vi "Close Hardware.vi"(8 "error in (no error)":errorcluster, 11 "Instrument.Template in":refnum<class "Instrument.Framework-Template.lvclass">) -> (0 "error out":errorcluster, 3 "Instrument.Template out":refnum<class "Instrument.Framework-Template.lvclass">)   [LabVIEW 2019, in "Instrument.Framework-Template.lvclass"]
uses:
  Instrument.Framework-Template.lvclass
  Instrument.Framework-Template.lvclass/Instrument.Framework-Template.ctl
  Framework/Instrument Types/SCPI/Instrument.SCPI.lvclass
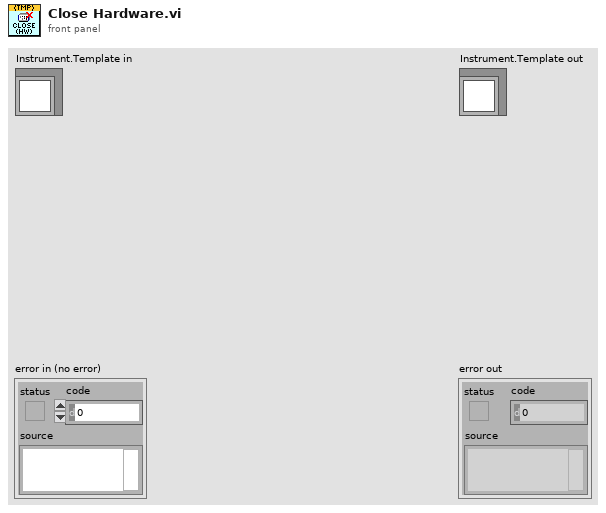
[diagram p1: front panel]
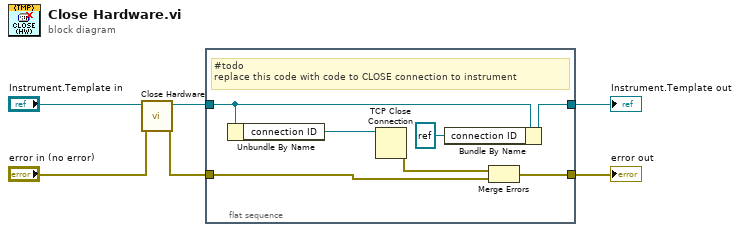
[diagram p0: block diagram]
diagram:
  n1 = call-parent "Close Hardware.vi"("error in (no error)"="error in (no error)", "Instrument in"="Instrument.Template in") -> ("error out"=w4:errorcluster, "Instrument out"=w2:refnum<class "Instrument.Framework-Template.lvclass">)  [unwired: 8 in]
  n2 = flat-sequence {
    tunnel: w4 -> [w9]
    tunnel: [w7] -> w3
    tunnel: w2 -> [w11]
    tunnel: [w10] -> w1
    frame #0 {
      # "#todo\nreplace this code with code to CLOSE connection to instrument"
      n3 = Unbundle By Name(w11) -> ("connection ID"=w13:refnum<k5>)
      n4 = TCP Close Connection(connection ID=w13) -> (error out=w8:errorcluster)  [unwired: 2 in, 1 out]
      n5 = Bundle By Name(cluster=w11, "connection ID"=refnum<k5> refnum) -> (w10:refnum<class "Instrument.Framework-Template.lvclass">)
      n6 = Merge Errors(w8, w9) -> (w7:errorcluster)
    }
  }
  "error out" <- w3
  "Instrument.Template out" <- w1
